vi "WSVCAP SHL Host TL RFFE Write - Multiple DUTs - Common Data.vi"(0 "Data Out":string, 11 "error in":errorcluster, 13 "DUT Mask (All)":bool[](array[boolean])=[TRUE, TRUE, TRUE, TRUE, TRUE, TRUE, TRUE, TRUE, TRUE, TRUE, TRUE, TRUE, TRUE, TRUE, TRUE, TRUE]) -> (15 "error out":errorcluster)   [LabVIEW 2012]
panel:
  out "Socket Mask":u16=1 format="%02x"
  out "SPI Data Out [U8]":u8[][](array[numeric]) format="%02x"
  # "DUT 01"
  # "DUT 02"
  # "DUT 03"
  # "DUT 04"
  # "DUT 05"
  # "DUT 06"
  # "DUT 07"
  # "DUT 08"
  # "DUT 09"
  # "DUT 10"
  # "DUT 11"
  # "DUT 12"
  # "DUT 13"
  # "DUT 14"
  # "DUT 15"
  # "DUT 16"
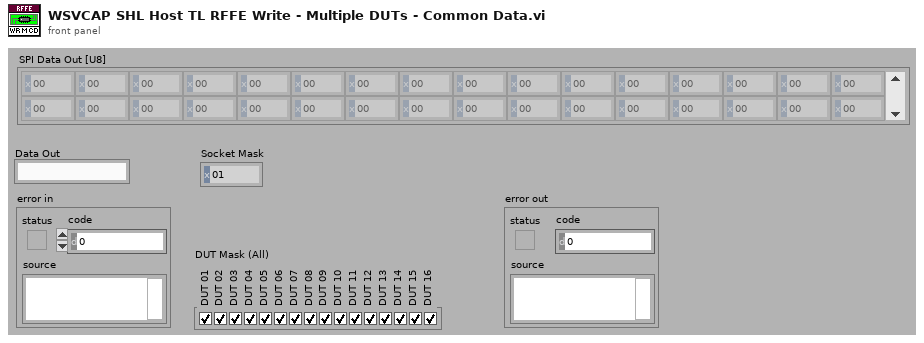
[diagram p1: front panel]
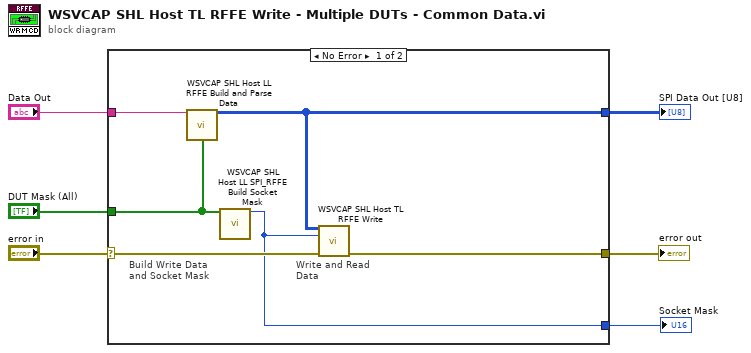
[diagram p0: block diagram]
diagram:
  n1 = case shown="No Error" "error in" {
    selector: "error in" -> [w11 _]
    tunnel: [w12 _] -> w6
    tunnel: "Data Out" -> [w10 _]
    tunnel: [w8 _] -> w3
    tunnel: [w7 _] -> w2
    tunnel: "DUT Mask (All)" -> [w9 _]
    frame No Error {
      # "Write and Read\nData"
      # "Build Write Data and Socket Mask"
      n2 = call "WSVCAP SHL Host LL RFFE Build and Parse Data.vi"("Data Out"=w10, "DUT Mask (All)"=w9) -> ("RFFE Data Out [U8]"=w8:u8[][])  [unwired: 10 in, 3 out]
      n3 = call "WSVCAP SHL Host LL SPI_RFFE Build Socket Mask.vi"("DUT Mask"=w9) -> ("Socket Mask [U16]"=w7:u16)  [unwired: 13 in, 1 out]
      n4 = call "WSVCAP SHL Host TL RFFE Write.vi"("RFFE Data Out"=w8, "Socket Mask"=w7, "error in"=w11) -> ("error out"=w12:errorcluster)  [unwired: 12 in]
    }
    frame Error {
    }
  }
  "error out" <- w6
  "SPI Data Out [U8]" <- w3
  "Socket Mask" <- w2
